vi "Write Full Module Name.vi"(8 "error in (no error)":errorcluster, 10 "Full Module Name":string, 11 "JSON Routing Channel Template in":refnum<class "JSON Routing Channel Template.lvclass">) -> (0 "error out":errorcluster, 3 "JSON Routing Channel Template out":refnum<class "JSON Routing Channel Template.lvclass">)   [LabVIEW 2020, in "Routing Templates.lvlib" / "JSON Routing Channel Template.lvclass"]
uses:
  JSON Routing Channel Template.lvclass
  JSON Routing Channel Template.lvclass/JSON Routing Channel Template.ctl
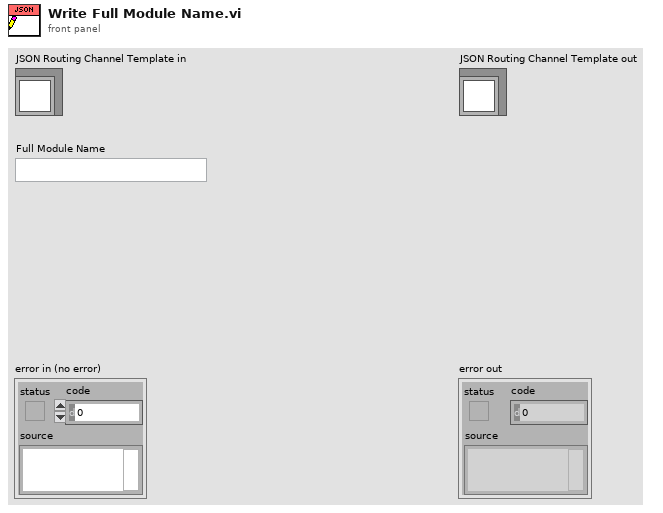
[diagram p1: front panel]
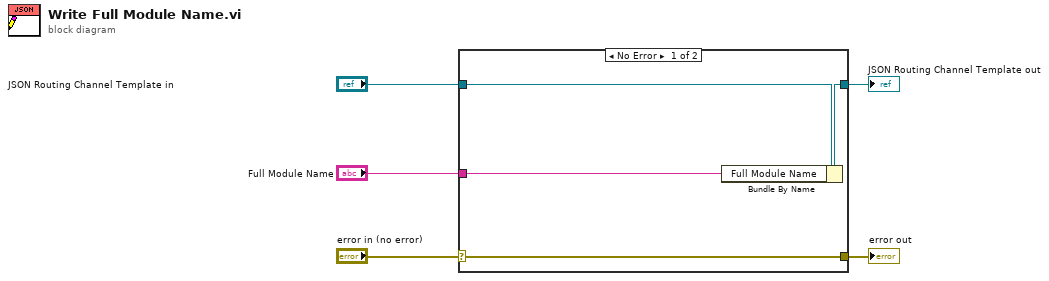
[diagram p0: block diagram]
diagram:
  n1 = case shown="No Error" "error in (no error)" {
    selector: "error in (no error)" -> [w9 w10]
    tunnel: [w9 w10] -> w4
    tunnel: [w7 w11] -> w2
    tunnel: "JSON Routing Channel Template in" -> [w8 w11]
    tunnel: "Full Module Name" -> [w6 _]
    frame No Error {
      n2 = Bundle By Name(cluster=w8, "Full Module Name"=w6) -> (w7:refnum<class "JSON Routing Channel Template.lvclass">)
    }
    frame Error {
    }
  }
  "error out" <- w4
  "JSON Routing Channel Template out" <- w2
